vi "LEP_RV_OnRun.vi"(8 "error in (no error)":errorcluster) -> (0 "error out":errorcluster)   [LabVIEW 2011]
doc: "Download and execute built VxWorks downloadable module and attach the LabVIEW Embedded debuger."
uses:
  LEP_RV_Commands.ctl
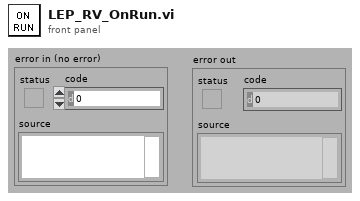
[diagram p1: front panel]
types:
  T1 = typedef "LEP_RV_Commands.ctl" = enum16{"Build", "Rebuild", "Run", "Debug", "Profile"}
  T2 = typedef "LEP_RV_Config.ctl" = cluster{"Enable debugging":bool, "Debug Options":u16, "Use stack variables":bool, "Generate serial only":bool, "Generate guard code":bool, "Generate Integer Only":bool, "Generate C Function Calls":bool, "ExpressionFolding":bool, "Constant Allocation":u16, "Constant Deallocation":u16, "Build Specification ID":string, "Preprocessor symbols (define)":string, "Compiler Flags":string, "Linker Flags":string, "Mode":u16, "Optimization":u16, "Optimize for time":bool, "Enable cross-module optimization":bool, "Include paths":path[], "Optimize heap size":bool, "Use MicroLib":bool, "Debug Mode":u16, "Enable profile information":bool, "Host name":string, "Use DHCP":bool, "IP address":string, "Subnet mask":string, "Gateway":string, "Primary DNS":string, "Secondary DNS":string, "MAC in target memory":bool, "MAC address":string, "Console output":u16, "Target serial port":u16}
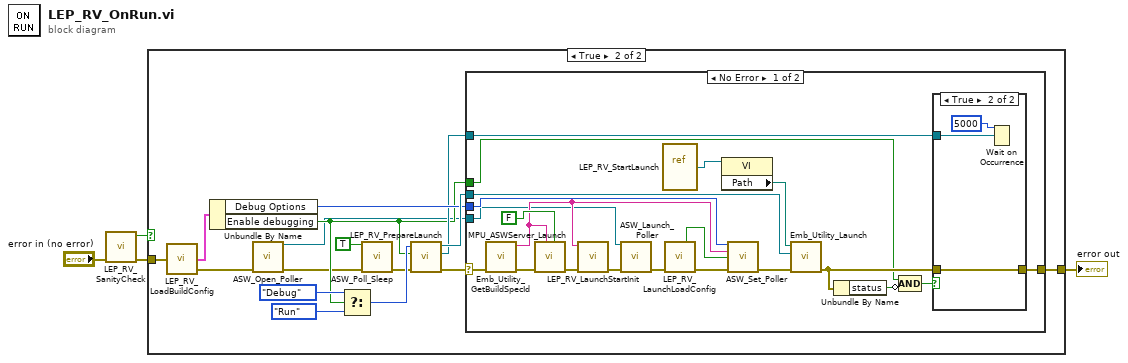
[diagram p0: block diagram]
diagram:
  n1 = call "LEP_RV_SanityCheck.vi"("error in (no error)"="error in (no error)") -> ("error out"=w2:errorcluster, "ok"=w1:bool)  [unwired: 1 in, 8 out]
  n2 = case shown="True" w1 {
    tunnel: [w5 w6] -> w3
    tunnel: w2 -> [w5 w7]
    frame False {
    }
    frame True {
      n3 = call "LEP_RV_LoadBuildConfig.vi"("error in (no error)"=w7) -> ("Config"=w17:T2, "error out"=w12:errorcluster)  [unwired: 1 out]
      n4 = Unbundle By Name(w17) -> ("Debug Options"=w16:u16, "Enable debugging"=w13:bool)
      n5 = call <vilib>:"ASW_Open_Poller.vi"("error in (no error)"=w12) -> ("vi reference"=w9:refnum<vi>, "error out"=w11:errorcluster)  [unwired: 13 in]
      n6 = Select(t=LEP_RV_Commands."Debug" ("Commands"), s=w13, f=LEP_RV_Commands."Run" ("Commands")) -> (s? t:f=w15:T1)
      n7 = call <vilib>:"ASW_Poll_Sleep.vi"("Sleep"=TRUE, "error in (no error)"=w11) -> ("error out"=w8:errorcluster)  [unwired: 13 in]
      n8 = call "LEP_RV_PrepareLaunch.vi"("error in (no error)"=w8, "Enable debugging"=w13, "Commands"=w15) -> ("error out"=w21:errorcluster, "debug occurrence"=w14:refnum<k4>, "output cluster"=w20:refnum<vi>)  [unwired: 6 in]
      n9 = case shown="No Error" w21 {
        selector: w21 -> [w39 w47]
        tunnel: [w34 w47] -> w6
        tunnel: w20 -> [w38 _]
        tunnel: w16 -> [w35 _]
        tunnel: w14 -> [w33 _]
        tunnel: w13 -> [w28 _]
        tunnel: w9 -> [w25 _]
        frame No Error {
          n10 = call <vilib>:"Emb_Utility_GetBuildSpecId.vi"("error in (no error)"=w39) -> ("error out"=w40:errorcluster, "buildSpec ID"=w31:string)  [unwired: 7 out]
          n11 = call <vilib>:"MPU_ASWServer_Launch.vi"("initialize (T)"=FALSE, "buildSpec ID"=w31, "error in"=w40) -> ("error out"=w32:errorcluster)  [unwired: 8 out]
          n12 = call "LEP_RV_LaunchStartInit.vi"("error in (no error)"=w32, "buildSpec ID"=w31) -> ("error out"=w30:errorcluster)  [unwired: 9 in]
          n13 = call <vilib>:"ASW_Launch_Poller.vi"("reference"=w25, "error in (no error)"=w30) -> ("error out"=w24:errorcluster)  [unwired: 13 in]
          n14 = vi-ref "LEP_RV_StartLaunch.vi"() -> (w42:refnum<vi>)
          n15 = call "LEP_RV_LaunchLoadConfig.vi"("error in (no error)"=w24) -> ("Connect to a network compile server"=w22:bool, "error out"=w23:errorcluster)  [unwired: 7 in, 6 out]
          n16 = property class="VI"(reference=w42) -> ("Path"=w41:path)  [unwired: 1 in, 2 out]
          n17 = call <vilib>:"ASW_Set_Poller.vi"("Debug Options"=w35, "buildSpec ID"=w31, "Connect to a network compile server"=w22, "error in (no error)"=w23) -> ("error out"=w36:errorcluster)  [unwired: 11 in]
          n18 = call <vilib>:"Emb_Utility_Launch.vi"("error in"=w36, "parameter cluster"=w38, "vi path"=w41) -> ("error out"=w29:errorcluster)  [unwired: 6 out]
          n19 = Unbundle By Name(w29) -> ("status"=w27:bool)
          n20 = Compound Arithmetic op=AND(w28, invert w27) -> (w26:bool)
          n21 = case shown="True" w26 {
            tunnel: w29 -> [w43 w45]
            tunnel: [w43 w45] -> w34
            tunnel: w33 -> [_ w44]
            frame False {
            }
            frame True {
              n22 = Wait on Occurrence(2:w44, 3:5000 ("ms timeout (-1)")) -> ()  [unwired: 1 in, 1 out]
            }
          }
        }
        frame Error {
        }
      }
    }
  }
  "error out" <- w3
